vi "rpTest.vi"(7 "LabVIEW Web Service Request Sp":refnum<class "Web Request.lvclass">, 8 "unit":dbl, 9 "targetPressure":dbl, 10 "maximumTolerance":dbl, 11 "minimumTolerance":dbl) -> (2 "current pr":dbl, 3 "maximumPressure":dbl format="%0.2f")   [LabVIEW 2015]
uses:
  <vilib>/wsapi/Web Request.lvclass
  Control test 1.ctl
  <vilib>/Waveform/WDTOps.llb/WDT Append Waveforms DBL.vi
panel:
  out "value":string
  in  "stop (F)":bool
  out "data":T1
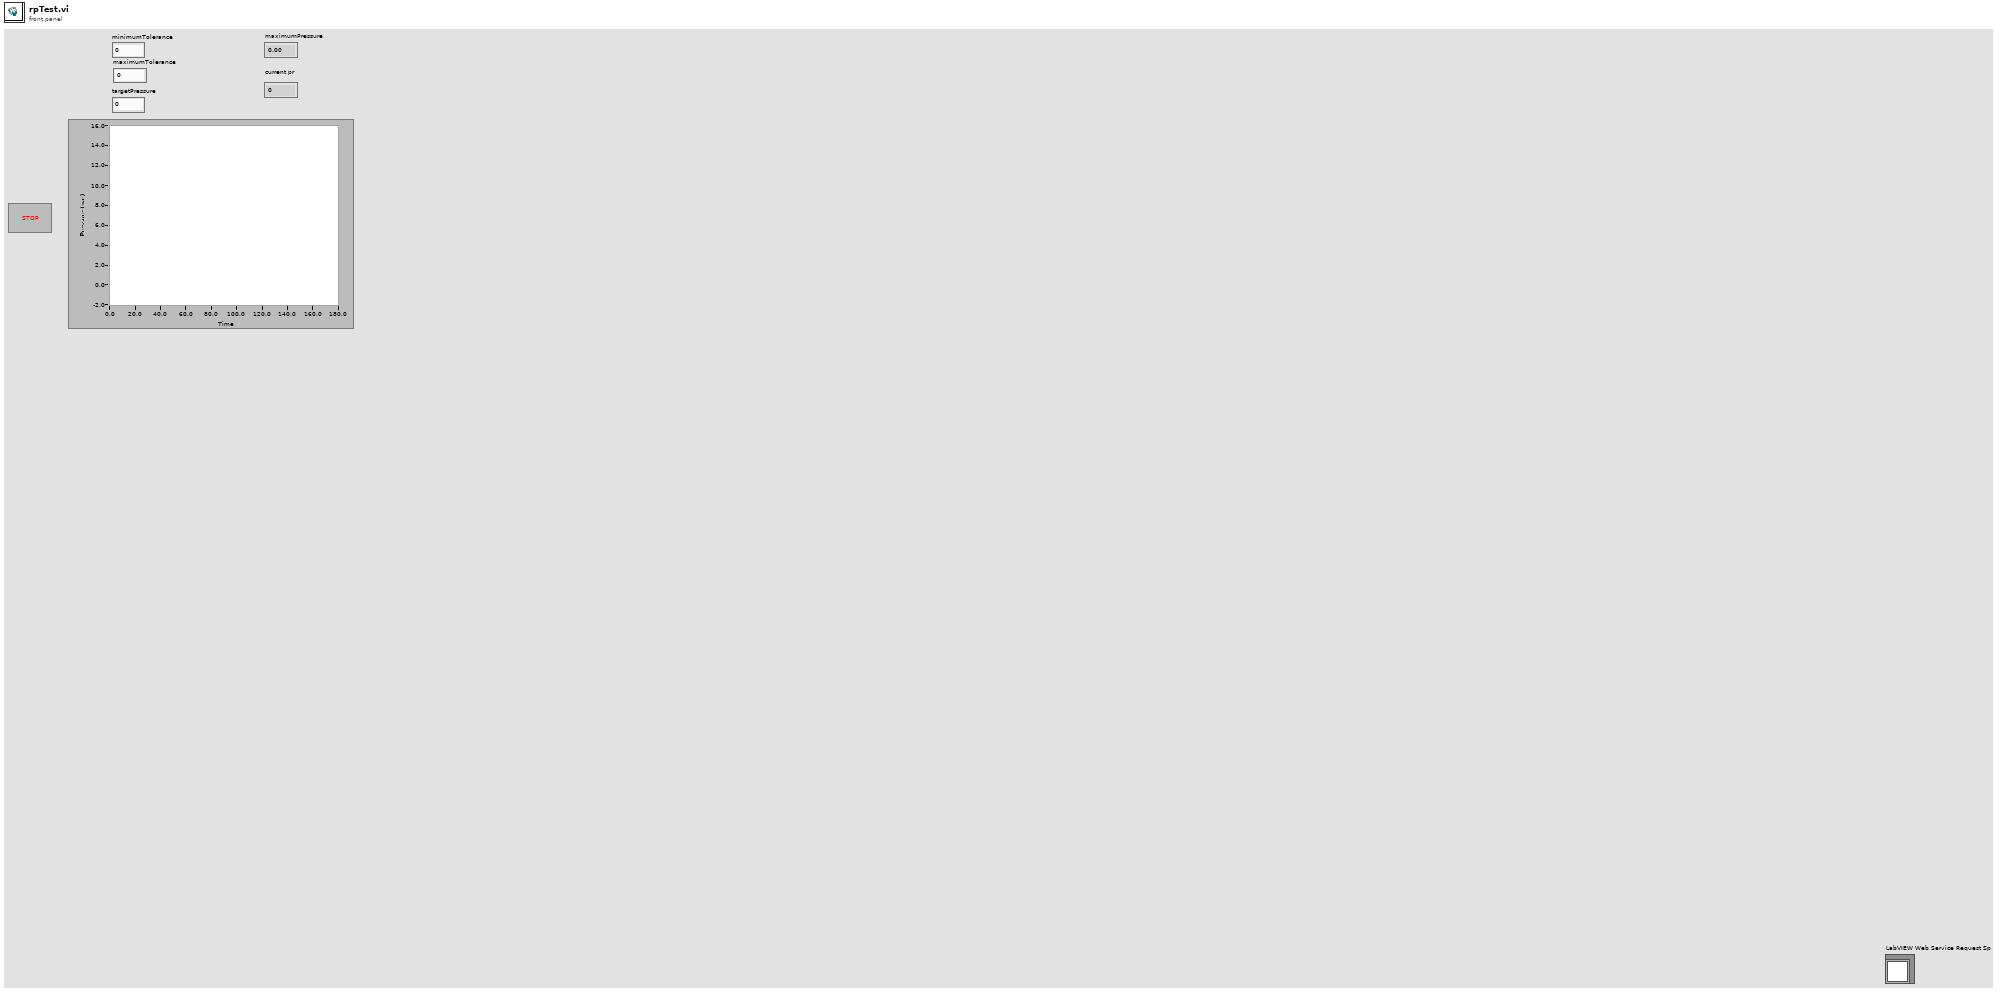
[diagram p1: front panel]
types:
  T1 = typedef "Control test 1.ctl" = dynamicdata
  T2 = typedef "imagedata.ctl" = cluster{"image type":i32, "image depth":i32, "image":u8[], "mask":u8[], "colors":u32[], "Rectangle":cluster{"left":i16, "top":i16, "right":i16, "bottom":i16}}
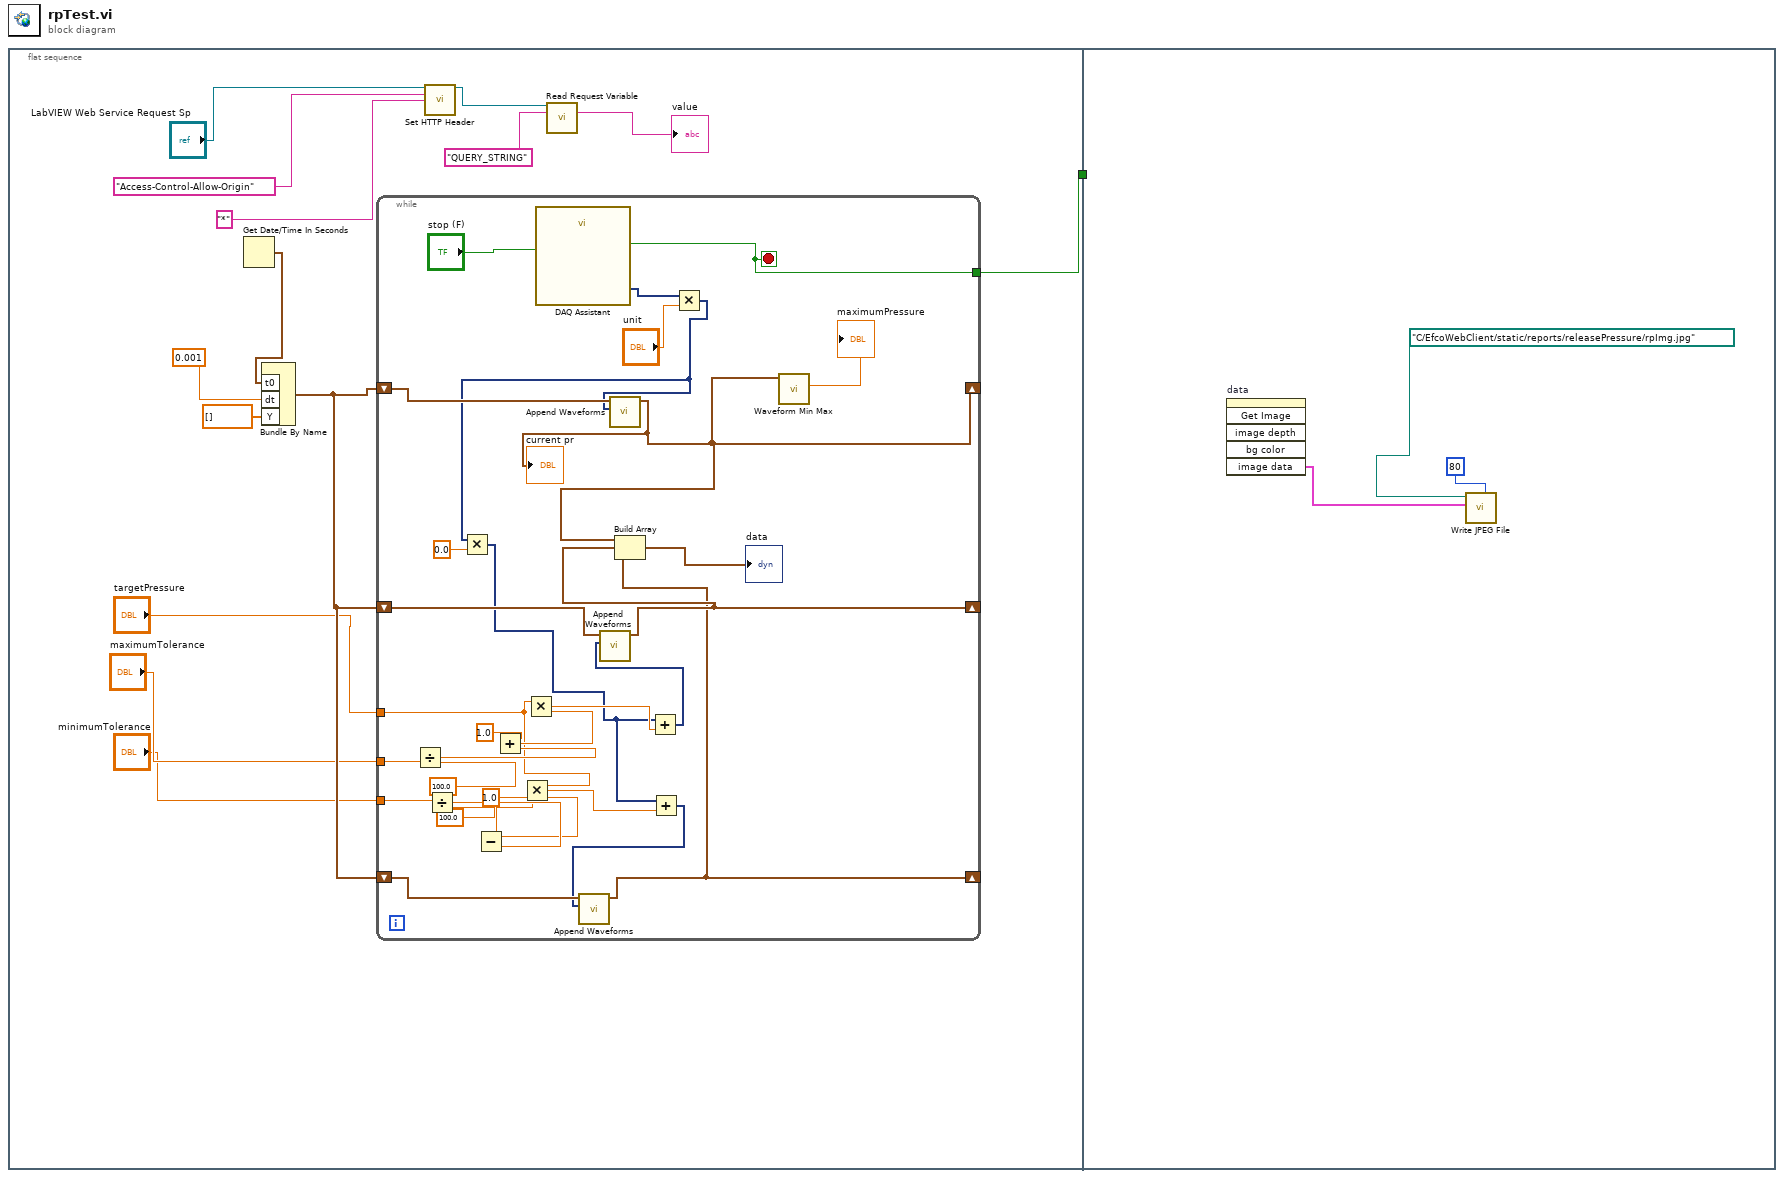
[diagram p0: block diagram]
diagram:
  n1 = flat-sequence {
    tunnel: [w8] -> w1
    tunnel: w1 -> [_]
    frame #0 {
      n2 = Get Date/Time In Seconds() -> (seconds since 1Jan1904=w14:timestamp)
      n3 = Bundle By Name("t0"=w14, "dt"=0.001, "Y"=dbl[] []) -> (w13:waveform(dbl))  [unwired: 1 in]
      n4 = while {
        shift-right: [w20] -> _
        shift-left: w13 -> [w23]
        shift-right: [w43] -> _
        shift-left: w13 -> [w44]
        tunnel: "maximumTolerance" -> [w42]
        tunnel: "minimumTolerance" -> [w40]
        tunnel: "targetPressure" -> [w32]
        shift-right: [w19] -> _
        shift-left: w13 -> [w28]
        tunnel: [w17] -> w8
        stop <- w17 stop-if-true
        n5 = Divide(x=w42, y=100.0) -> (x/y=w37:dbl)
        n6 = Divide(x=w40, y=100.0) -> (x/y=w36:dbl)
        n7 = Subtract(x=1.0, y=w36) -> (x-y=w34:dbl)
        n8 = Add(x=1.0, y=w37) -> (x+y=w33:dbl)
        n9 = Multiply(x=w32, y=w34) -> (x*y=w26:dbl)
        n10 = Multiply(x=w32, y=w33) -> (x*y=w30:dbl)
        n11 = call "DAQ Assistant"("stop (F)"="stop (F)") -> ("data"=w24:dynamicdata, "stopped"=w17:bool)  [unwired: 15 in, 2 out]
        n12 = Multiply(x=w24, y="unit") -> (x*y=w21:dynamicdata)
        n13 = Multiply(x=w21, y=0.0) -> (x*y=w27:dynamicdata)
        n14 = call-poly <vilib>:"Append Waveforms.vi"("waveform B"=w21, "waveform A"=w23) -> ("waveform out"=w20:waveform(dbl))  [unwired: 8 in, 1 out]
        "current pr" <- w20
        n15 = Add(x=w27, y=w30) -> (x+y=w29:dynamicdata)
        n16 = call-poly <vilib>:"Append Waveforms.vi"("waveform B"=w29, "waveform A"=w44) -> ("waveform out"=w43:waveform(dbl))  [unwired: 8 in, 1 out]
        n17 = Add(x=w27, y=w26) -> (x+y=w25:dynamicdata)
        n18 = call-poly <vilib>:"Append Waveforms.vi"("waveform B"=w25, "waveform A"=w28) -> ("waveform out"=w19:waveform(dbl))  [unwired: 8 in, 1 out]
        n19 = Build Array(w20, w43, w19) -> (→"data":waveform(dbl)[])
        n20 = call <vilib>:"Waveform Min Max.vi"("waveform in"=w20) -> ("Y max"=→"maximumPressure":dbl)  [unwired: 5 in, 5 out]
      }
      n21 = call <vilib>:"Set HTTP Header.vi"("LabVIEW Web Service Request"="LabVIEW Web Service Request Sp", "header"="Access-Control-Allow-Origin", "header value"="*") -> ("LabVIEW Web Service Request out"=w4:refnum<class "Web Request.lvclass">)  [unwired: 11 in, 1 out]
      n22 = call <vilib>:"Read Request Variable.vi"("LabVIEW Web Service Request"=w4, "variable name"="QUERY_STRING") -> ("value"=→"value":string)  [unwired: 11 in, 2 out]
    }
    frame #1 {
      n23 = invoke on="data" class="WFGraph (strict)" method="Get Image"() -> ("image data"=w48:T2)  [unwired: 6 in, 5 out]
      n24 = call <vilib>:"Write JPEG File.vi"("quality (80)"=80, "image data"=w48, "path to JPEG file"=path "C:/EfcoWebClient/static/reports/releasePressure/rpImg.jpg") -> ()  [unwired: 7 in, 2 out]
    }
  }
